vi "Demo of DBSCAN clustering.vi"() -> ()   [LabVIEW 2020]
doc: "Finds core samples of high density and expands clusters from them."
uses:
  Model/Unsupervised/Cluster/DBSCAN/Controls/dbscan_params.ctl
  Display/_Controls/Style.ctl
  Display/Classification/2D/Predicted/Controls/PredictedParameter.ctl
  Model/Unsupervised/Cluster/DBSCAN/DBSCAN.lvclass
  C:/Users/cipop/TDF Dropbox/2_Technologies de France/1 - Services et Etudes/PLAIY/2 - DEV/PLAIYLAB/code/Model/Model.lvclass
  Model/Unsupervised/Cluster/DBSCAN/DBSCAN.vi
  Preproc/Objet/3 - Model selection and evaluation/3.3 - Metrics and scoring/homogeneity_score/Homogeneity_Score.vi
  Preproc/Objet/3 - Model selection and evaluation/3.3 - Metrics and scoring/completeness_score/Completeness_Score.vi
  Preproc/Objet/3 - Model selection and evaluation/3.3 - Metrics and scoring/v_measure_score/V_Measure_Score.vi
  Preproc/Objet/3 - Model selection and evaluation/3.3 - Metrics and scoring/adjusted_rand_score/Adjusted_Rand_Score.vi
  Preproc/Objet/3 - Model selection and evaluation/3.3 - Metrics and scoring/adjusted_mutual_info_score/Adjusted_Mutual_Info_Score.vi
  Preproc/Objet/3 - Model selection and evaluation/3.3 - Metrics and scoring/silhouette_score/Silhouette_Score.vi
  Preproc/Objet/6 - Datasets Transformation/6.3 - Processing Data/StandardScaler/StandardScaler.lvclass
panel:
  in  "Local":T1
  in  "error in (no error) 2":errorcluster caption="entrée d'erreur (pas d'erreur)"
  out "Plot 2":cluster{"X":dbl[], "Y":dbl[]}[](graph) caption="Estimated number of cluster: 3"
  out "class_member_mask":bool[][](array[boolean])
  out "~core_samples_mask":bool[](array[boolean])
  out "n_noise_":i32
  out "error out":errorcluster
  out "Plot":cluster{"X":dbl[], "Y":dbl[]}[](graph) caption="Estimated number of cluster: 3"
  out "Silhouette Coefficient":string
  out "Adjusted Mutual Information":string
  out "Adjusted Rand Index":string
  out "V-measure":string
  out "Completeness":string
  out "Homogeneity":string
  out "n_clusters_":i32
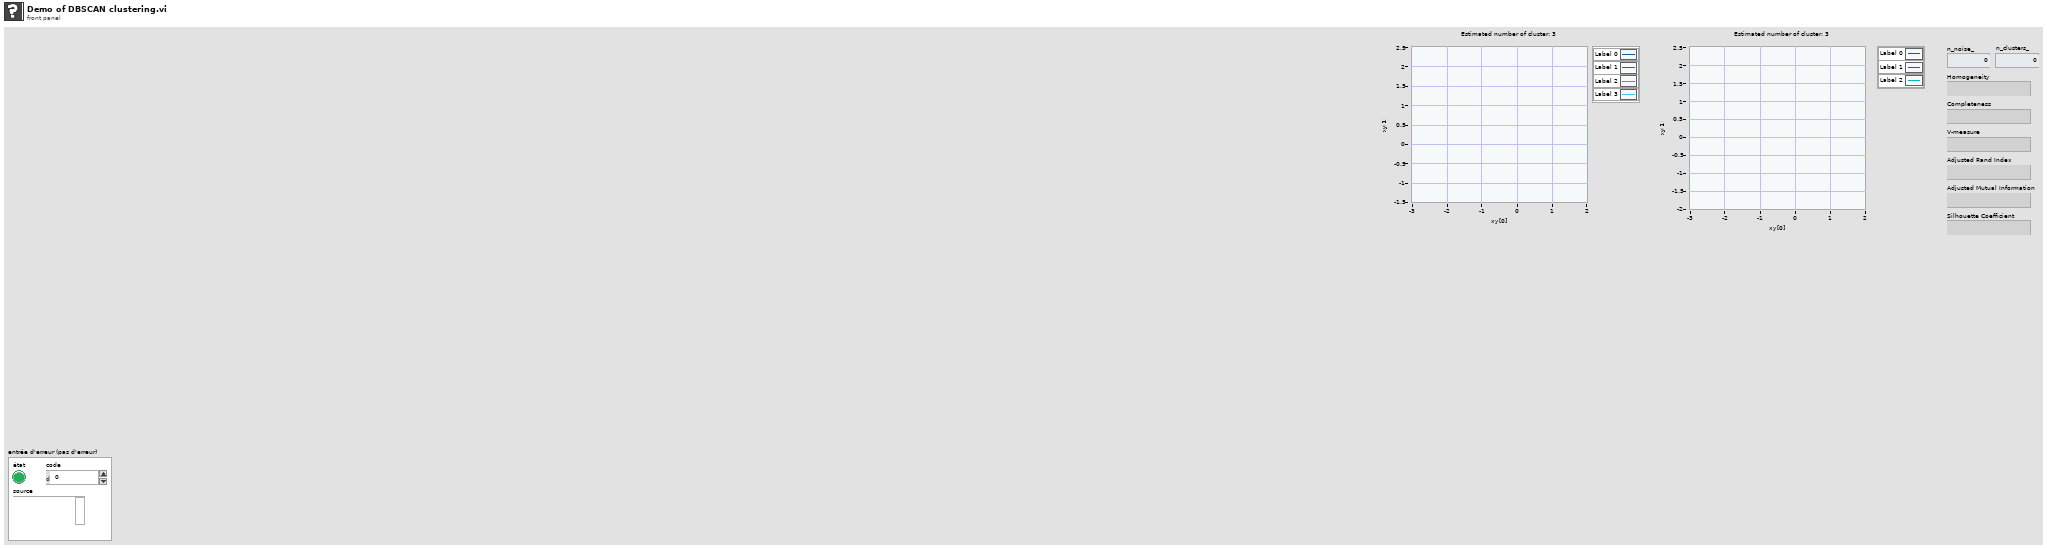
[diagram p1: front panel]
types:
  T1 = cluster{"X":dbl[][], "labels_true":dbl[], "core_sample_indices_":dbl[], "labels_":dbl[], "core_samples_mask":bool[], "Set_Label":dbl[], "1_Add_Mask":dbl[][], "2_Add_Mask":dbl[][], "1_Label_Add_Mask":dbl[][], "2_Label_Add_Mask":dbl[][]}
  T2 = cluster{"copy":bool, "with_mean":bool, "with_std":bool}
  T3 = cluster{"n_samples":i32[], "n_features":u32, "centers":i32[][], "cluster_std":dbl[], "centermin":dbl, "centermax":dbl, "shuffle":bool, "random_state":i32, "Returns":string}
  T4 = typedef "dbscan_params.ctl" = cluster{"eps":dbl, "min_samples":dbl, "metric":string, "algorithm":string, "leaf_size":dbl, "p":dbl, "n_jobs":dbl}
  T5 = typedef "Style.ctl" = enum16{"Empty circle", "Full circle", "Empty square", "Full square", "Cross"}
  T6 = typedef "PredictedParameter.ctl" = cluster{"Plot":refnum<vi>, "Data":cluster{"X":dbl[][], "Predict":dbl[][]}, "Indexe":cluster{"X":i32, "Y":i32}, "Point Property":cluster{"Style":T5, "Label Color":u32[]}}
  T7 = cluster{" 4DArray":cluster{"1":string[][], "2":string[][]}[], " 3DArray":cluster{"Tableau":string[][]}[], "Sparse Matrix 2DArray":string[][], " 2DArray":string[][], " 1DArray":string[]}
  T8 = typedef "dbscan_attributes.ctl" = cluster{"core_sample_indices_":dbl[], "components_":dbl[][], "labels_":dbl[]}
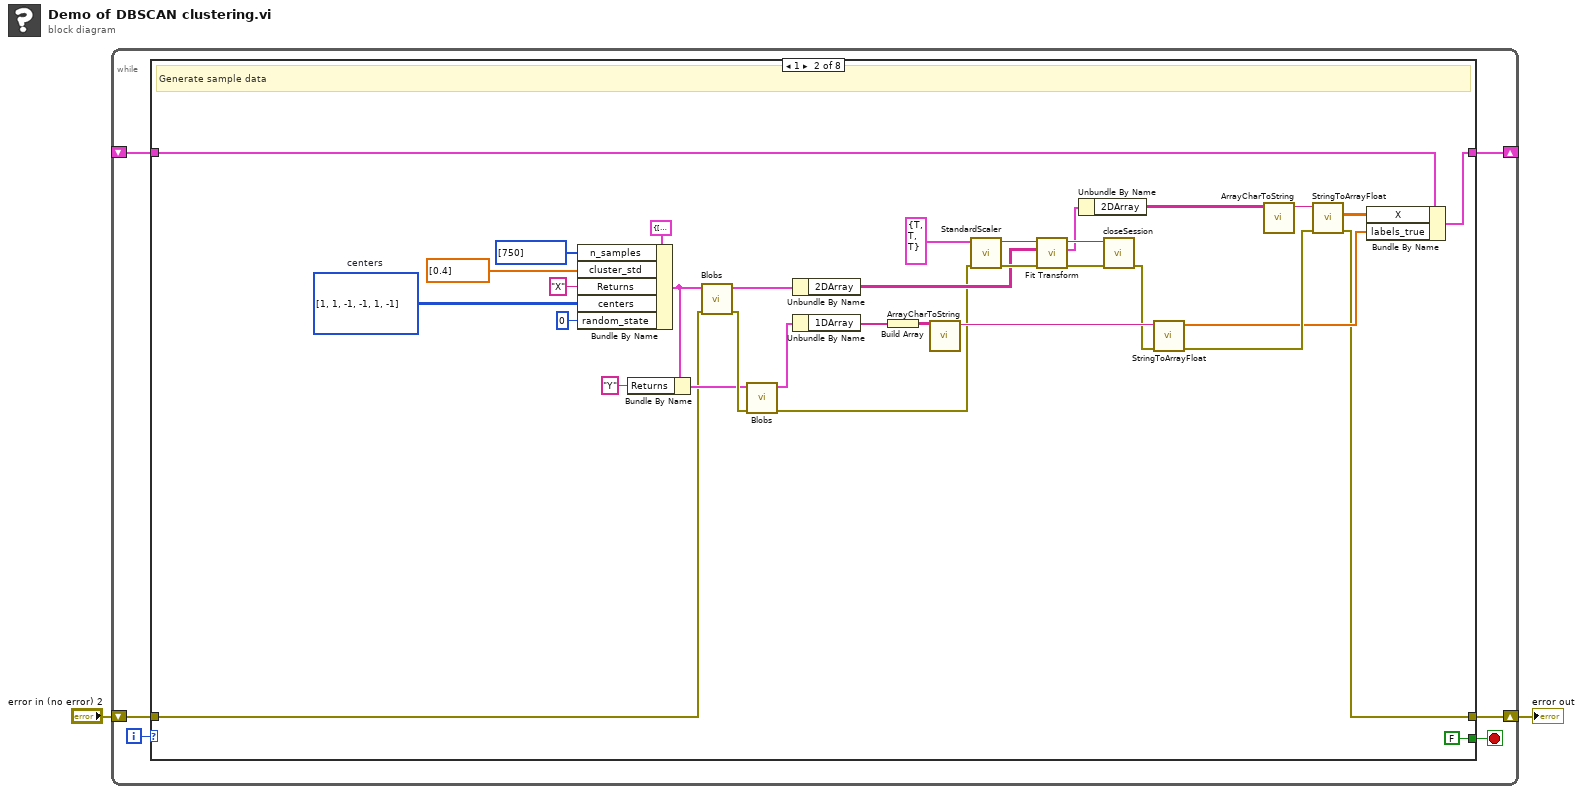
[diagram p0: block diagram]
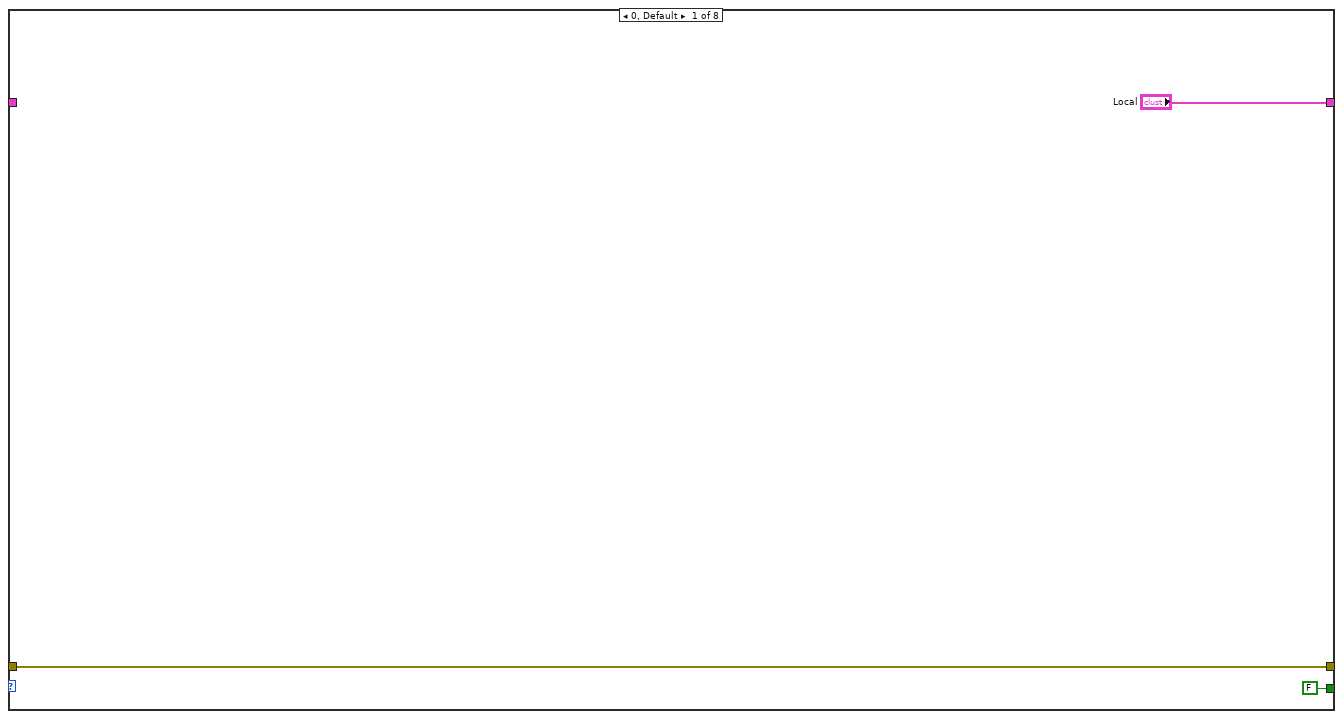
[diagram p2: hidden frame]
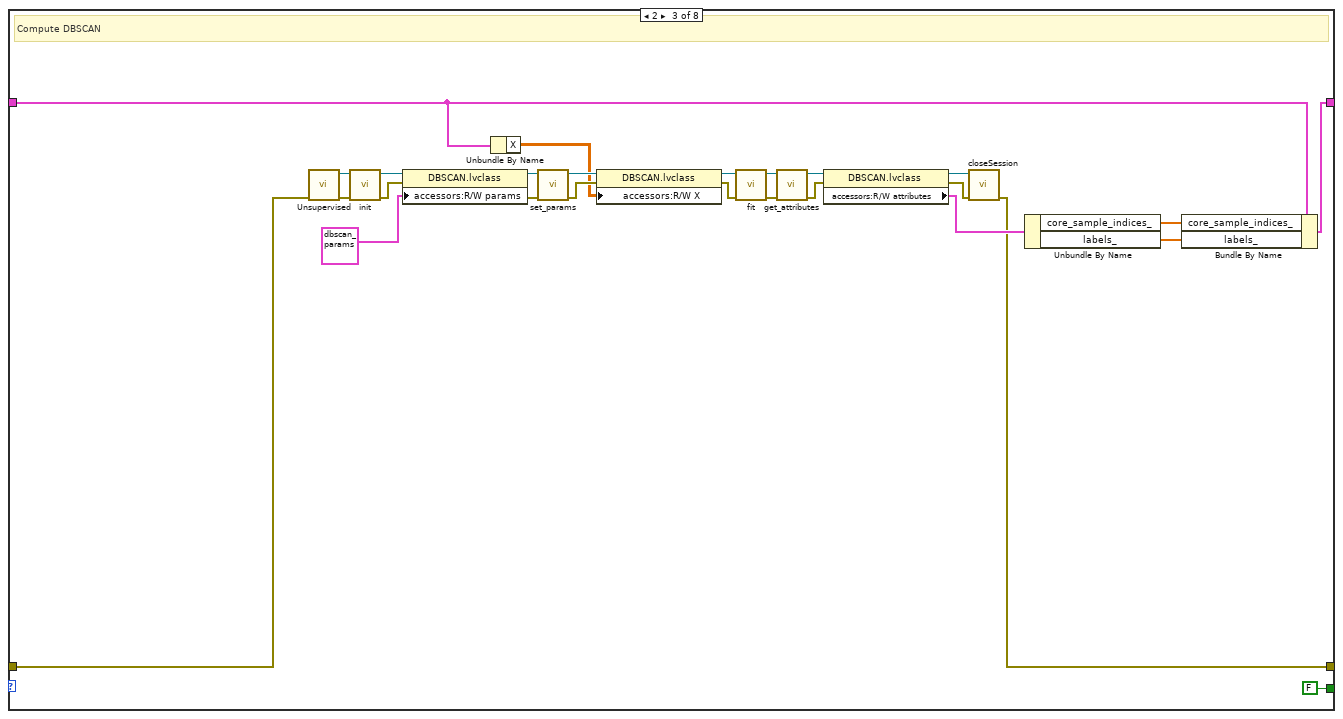
[diagram p3: hidden frame]
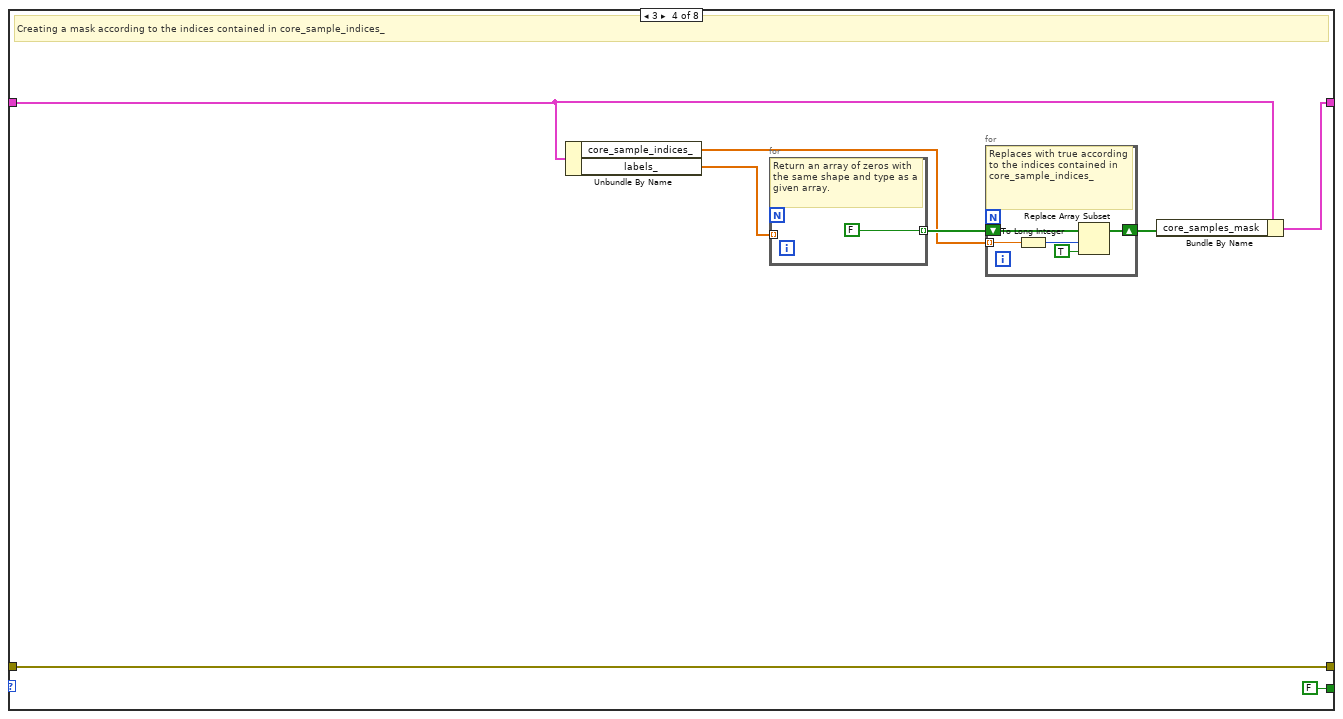
[diagram p4: hidden frame]
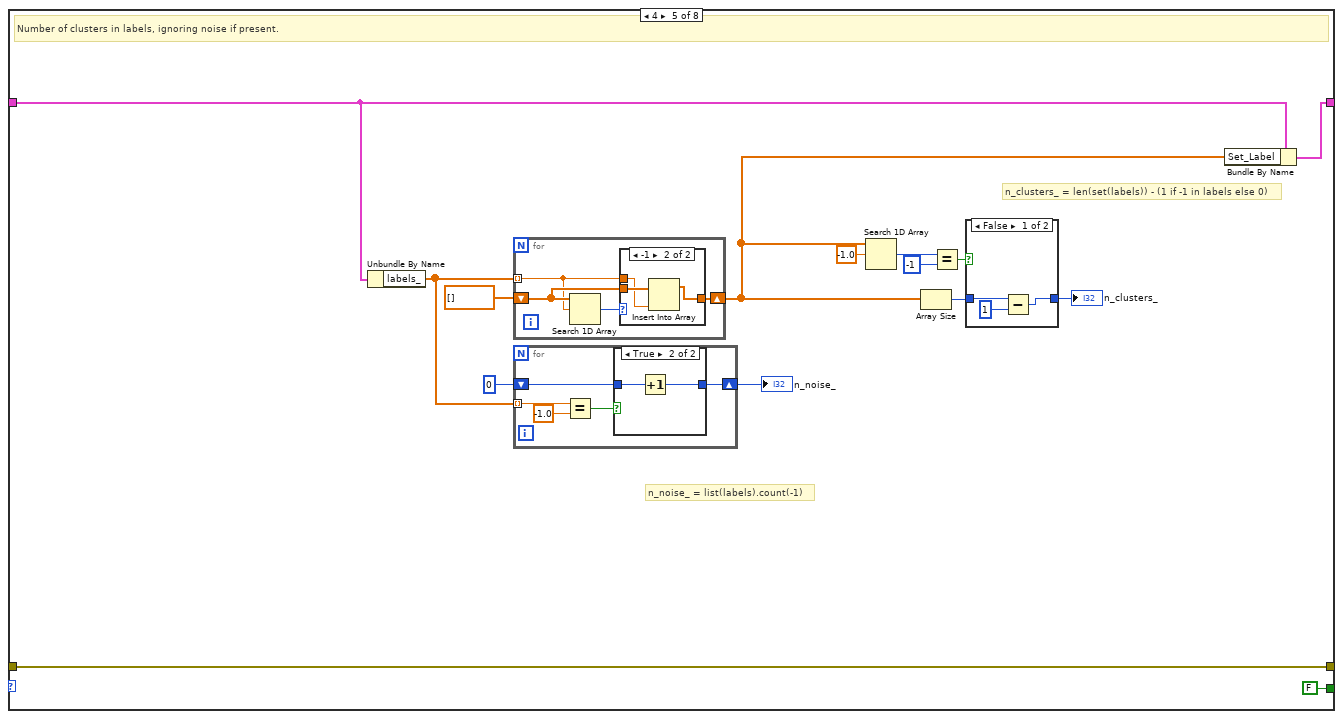
[diagram p5: hidden frame]
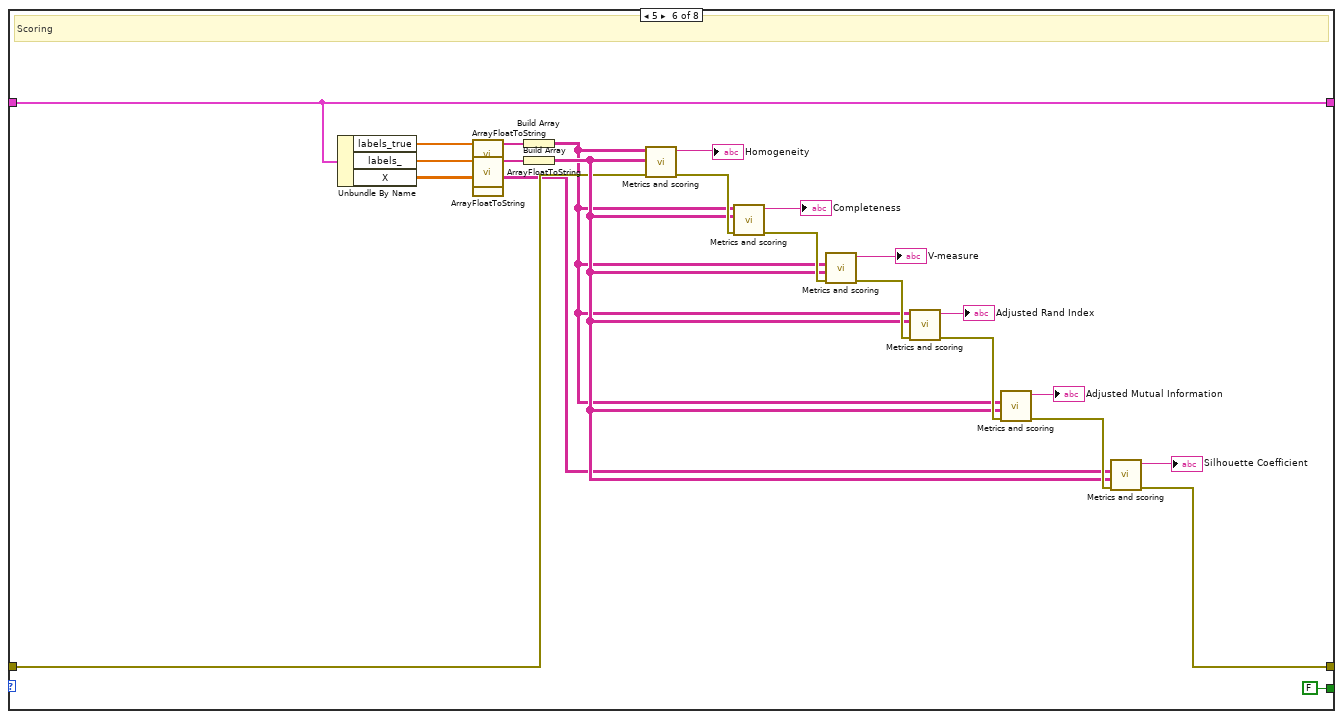
[diagram p9: hidden frame]
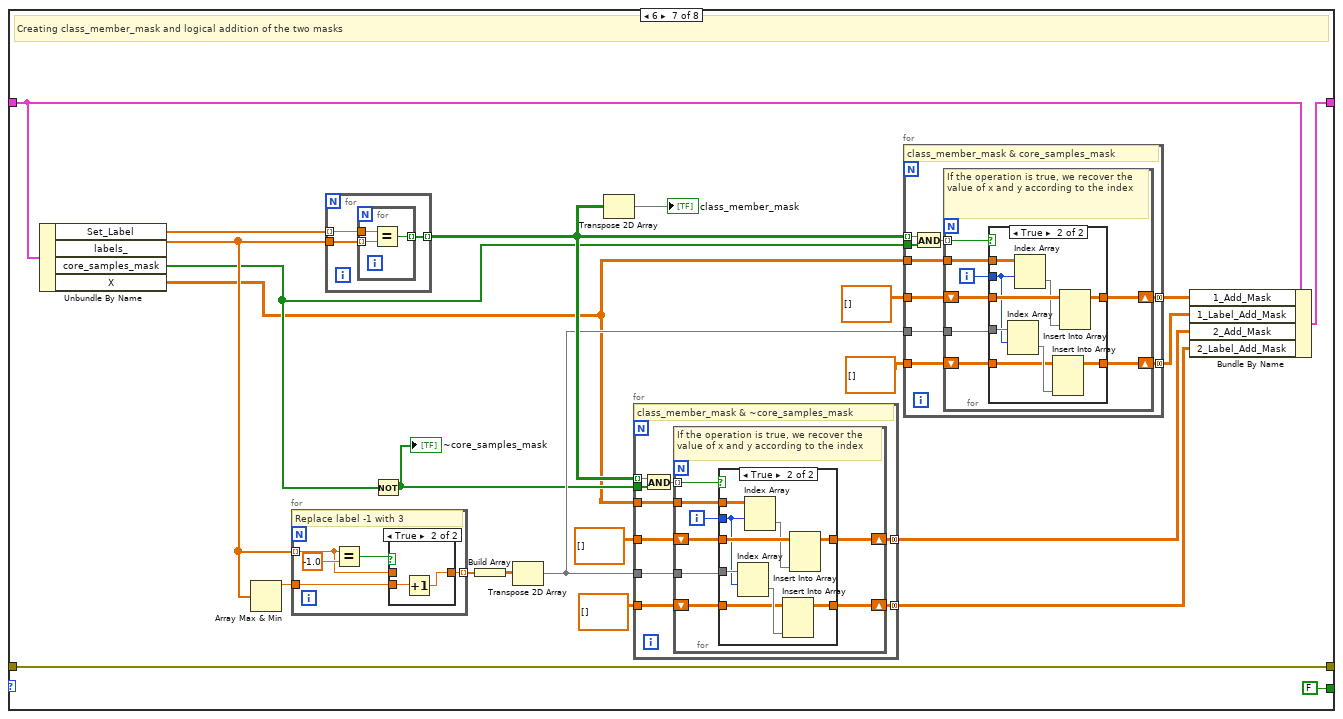
[diagram p10: hidden frame]
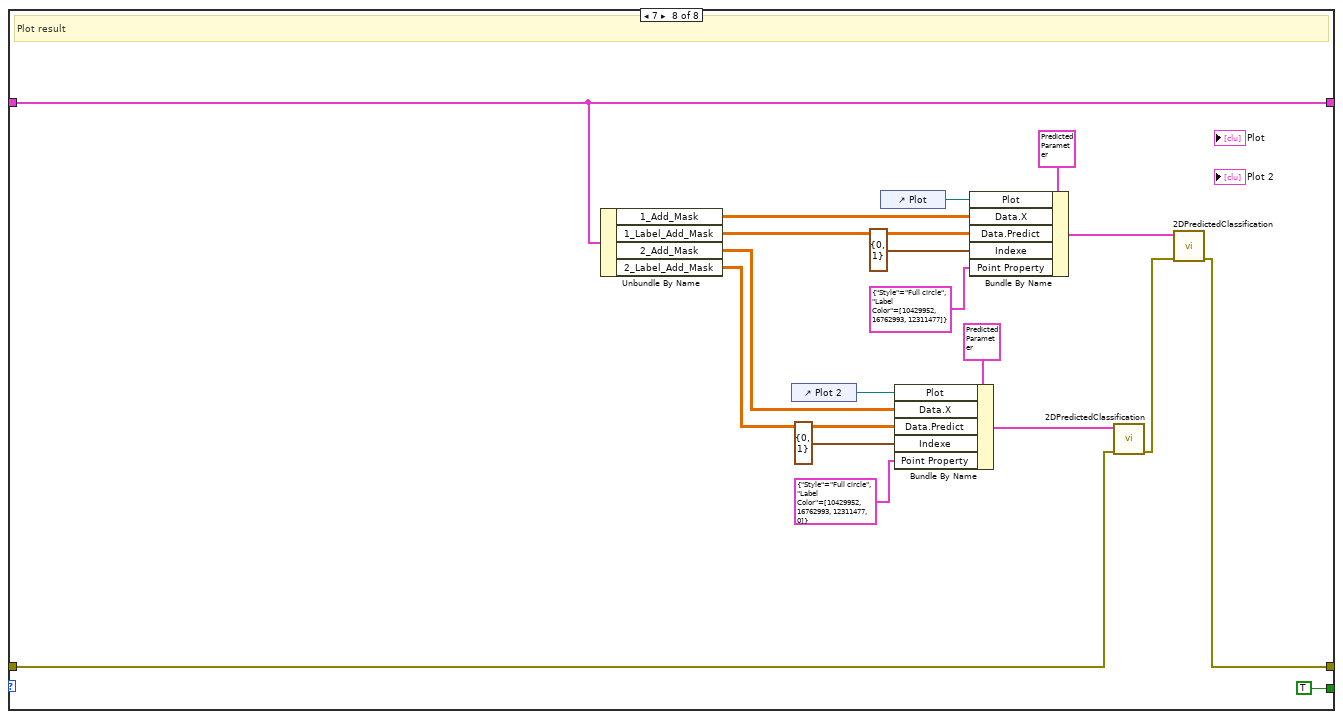
[diagram p14: hidden frame]
diagram:
  n1 = while {
    shift-right: [w3] -> _
    shift-left: _ -> [w7]
    shift-right: [w5] -> w1
    shift-left: "error in (no error) 2" -> [w6]
    i -> [w8]
    stop <- w4 stop-if-true
    n2 = case shown="1" w8 {
      tunnel: ["Local" w17 w53 w77 w93 w129 w150 w242] -> w3
      tunnel: w7 -> [_ w18 w49 w76 w88 w129 w151 w242]
      tunnel: w6 -> [w11 w13 w47 w73 w91 w127 w145 w245]
      tunnel: [w11 w14 w50 w73 w91 w136 w145 w246] -> w5
      tunnel: [FALSE FALSE FALSE FALSE FALSE FALSE FALSE TRUE] -> w4
      frame 0, Default {
      }
      frame 1 {
        w33 = i32[][] [[1, 1], [-1, -1], [1, -1]]  # centers
        # "Generate sample data"
        n3 = Bundle By Name(cluster=T3 {"n_samples"=[100], "n_features"=2, "centers"=[], "cluster_std"=[], "centermin"=-10.0, "centermax"=10.0, "shuffle"=TRUE, "random_state"=-1, "Returns"="X"} ("make_blobs"), "n_samples"=i32[] [750], "cluster_std"=dbl[] [0.4], "Returns"="X", "centers"=w33, "random_state"=0) -> (w31:T3)
        n4 = Bundle By Name(cluster=w31, "Returns"="Y") -> (w39:T3)
        n5 = call "Blobs.vi"("error in (no error)"=w13, "make_blobs"=w31) -> ("error out"=w43:errorcluster, "Data"=w45:T7)  [unwired: 8 in]
        n6 = call "Blobs.vi"("error in (no error)"=w43, "make_blobs"=w39) -> ("error out"=w23:errorcluster, "Data"=w38:T7)  [unwired: 8 in]
        n7 = Unbundle By Name(w45) -> ("2DArray"=w24:string[][])
        n8 = Unbundle By Name(w38) -> ("1DArray"=w35:string[])
        n9 = Build Array(w35) -> (w34:string[][])
        n10 = call "ArrayCharToString.vi"("TAB"=w34) -> ("Instruction"=w36:string)  [unwired: 10 in]
        n11 = call "StandardScaler.vi"("error in (no error)"=w23, "StandardScaler"=T2 {"copy"=TRUE, "with_mean"=TRUE, "with_std"=TRUE}) -> ("error out"=w25:errorcluster, "StandardScaler.lvclass"=w28:refnum<class "StandardScaler.lvclass">)  [unwired: 8 in]
        n12 = call-dynamic "Fit Transform.vi"("error in (no error)"=w25, "X"=w24, "StandardScaler.lvclass"=w28) -> ("error out"=w26:errorcluster, "Data"=w21:T7, "StandardScaler.lvclass"=w27:refnum<class "StandardScaler.lvclass">)  [unwired: 6 in]
        n13 = Unbundle By Name(w21) -> ("2DArray"=w20:string[][])
        n14 = call-dynamic "closeSession.vi"("error in"=w26, "Python en entrée"=w27) -> ("error out"=w22:errorcluster)  [unwired: 8 in, 1 out]
        n15 = call "StringToArrayFloat.vi"("entrée d'erreur (pas d'erreur)"=w22, "Return value"=w36) -> ("error IO"=w19:errorcluster, "1DArray"=w15:dbl[])  [unwired: 7 in, 1 out]
        n16 = call "ArrayCharToString.vi"("TAB"=w20) -> ("Instruction"=w44:string)  [unwired: 10 in]
        n17 = call "StringToArrayFloat.vi"("entrée d'erreur (pas d'erreur)"=w19, "Return value"=w44) -> ("error IO"=w14:errorcluster, "2DArray"=w16:dbl[][])  [unwired: 7 in, 1 out]
        n18 = Bundle By Name(cluster=w18, "X"=w16, "labels_true"=w15) -> (w17:T1)
      }
      frame 2 {
        # "Compute DBSCAN"
        n19 = call-poly "Unsupervised.vi"("error in"=w47) -> ("error out"=w70:errorcluster, "out"=w71:refnum<class "DBSCAN.lvclass">)  [unwired: 9 in]
        n20 = call-dynamic "init.vi"("error in (no error)"=w70, "Model en entrée"=w71) -> ("error out"=w62:errorcluster, "Model en sortie"=w66:refnum<class "DBSCAN.lvclass">)  [unwired: 8 in]
        n21 = property class="DBSCAN.lvclass"(reference=w66, error in=w62, "accessors:R/W params"=T4 {"eps"=0.3, "min_samples"=10.0, "metric"="euclidean", "algorithm"="auto", "leaf_size"=30.0, "p"=2.0, "n_jobs"=1.0} ("R/W params")) -> (reference out=w65:refnum<class "DBSCAN.lvclass">, error out=w67:errorcluster)
        n22 = Unbundle By Name(w49) -> ("X"=w48:dbl[][])
        n23 = call-dynamic "set_params.vi"("error in (no error)"=w67, "DBSCAN.lvclass 2"=w65) -> ("error out"=w63:errorcluster, "DBSCAN.lvclass"=w64:refnum<class "DBSCAN.lvclass">)  [unwired: 8 in]
        n24 = property class="DBSCAN.lvclass"(reference=w64, error in=w63, "accessors:R/W X"=w48) -> (reference out=w69:refnum<class "DBSCAN.lvclass">, error out=w68:errorcluster)
        n25 = call-dynamic "fit.vi"("error in (no error)"=w68, "DBSCAN.lvclass 2"=w69) -> ("error out"=w58:errorcluster, "DBSCAN.lvclass"=w59:refnum<class "DBSCAN.lvclass">)  [unwired: 8 in]
        n26 = call-dynamic "get_attributes.vi"("error in (no error)"=w58, "DBSCAN.lvclass 2"=w59) -> ("error out"=w56:errorcluster, "DBSCAN.lvclass"=w57:refnum<class "DBSCAN.lvclass">)  [unwired: 8 in]
        n27 = property class="DBSCAN.lvclass"(reference=w57, error in=w56) -> (reference out=w61:refnum<class "DBSCAN.lvclass">, error out=w60:errorcluster, "accessors:R/W attributes"=w55:T8)
        n28 = call-dynamic "closeSession.vi"("error in"=w60, "Python en entrée"=w61) -> ("error out"=w50:errorcluster)  [unwired: 8 in, 1 out]
        n29 = Unbundle By Name(w55) -> ("core_sample_indices_"=w52:dbl[], "labels_"=w51:dbl[])
        n30 = Bundle By Name(cluster=w49, "core_sample_indices_"=w52, "labels_"=w51) -> (w53:T1)
      }
      frame 3 {
        # "Creating a mask according to the indices contained in core_sample_indices_"
        n31 = Unbundle By Name(w76) -> ("core_sample_indices_"=w75:dbl[], "labels_"=w74:dbl[])
        n32 = for {
          tunnel: [FALSE] -> w79 mode=indexing
          tunnel: w74 -> [_] mode=indexing
          # "Return an array of zeros with the same shape and type as a given array."
        }
        n33 = for {
          tunnel: w75 -> [w84] mode=indexing
          shift-right: [w80] -> w78
          shift-left: w79 -> [w83]
          # "Replaces with true according to the indices contained in core_sample_indices_"
          n34 = To Long Integer(number=w84) -> (32bit integer=w82:i32)
          n35 = Replace Array Subset(array=w83, new element=TRUE ("new element/subarray"), index=w82) -> (w80:bool[])
        }
        n36 = Bundle By Name(cluster=w76, "core_samples_mask"=w78) -> (w77:T1)
      }
      frame 4 {
        # "n_noise_ = list(labels).count(-1)"
        # "n_clusters_ = len(set(labels)) - (1 if -1 in labels else 0)"
        # "Number of clusters in labels, ignoring noise if present."
        n37 = Unbundle By Name(w88) -> ("labels_"=w87:dbl[])
        n38 = for {
          tunnel: w87 -> [w114] mode=indexing
          shift-right: [w113] -> w92
          shift-left: dbl[] [] ("labels_") -> [w115]
          n39 = Search 1D Array(1D array=w115, element=w114) -> (index of element=w116:i32)  [unwired: 1 in]
          n40 = case shown="-1" w116 {
            tunnel: w115 -> [w117 w120]
            tunnel: w114 -> [_ w119]
            tunnel: [w117 w118] -> w113
            frame Default {
            }
            frame -1 {
              n41 = Insert Into Array(array=w120, new element=w119) -> (w118:dbl[])  [unwired: 1 in]
            }
          }
        }
        n42 = for {
          tunnel: w87 -> [w105] mode=indexing
          shift-right: [w102] -> w89
          shift-left: 0 -> [w101]
          n43 = Equal?(x=w105, y=-1.0) -> (x = y?=w103:bool)
          n44 = case shown="True" w103 {
            tunnel: [w106 w108] -> w102
            tunnel: w101 -> [w106 w107]
            frame False {
            }
            frame True {
              n45 = Increment(x=w107) -> (x+1=w108:i32)
            }
          }
        }
        "n_noise_" <- w89
        n46 = Search 1D Array(1D array=w92, element=-1.0) -> (index of element=w99:i32)  [unwired: 1 in]
        n47 = Array Size(array=w92) -> (size(s)=w98:i32)
        n48 = Equal?(x=w99, y=-1) -> (x = y?=w100:bool)
        n49 = case shown="False" w100 {
          tunnel: w98 -> [w111 w112]
          tunnel: [w109 w112] -> w90
          frame False {
            n50 = Subtract(x=w111, y=1) -> (x-y=w109:i32)
          }
          frame True {
          }
        }
        "n_clusters_" <- w90
        n51 = Bundle By Name(cluster=w88, "Set_Label"=w92) -> (w93:T1)
      }
      frame 5 {
        # "Scoring"
        n52 = Unbundle By Name(w129) -> ("labels_true"=w125:dbl[], "labels_"=w128:dbl[], "X"=w123:dbl[][])
        n53 = call "ArrayFloatToString.vi"("1D Data"=w125) -> ("Array"=w126:string[])  [unwired: 9 in, 1 out]
        n54 = call "ArrayFloatToString.vi"("1D Data"=w128) -> ("Array"=w142:string[])  [unwired: 9 in, 1 out]
        n55 = call "ArrayFloatToString.vi"("2D Data"=w123) -> ("Array"=w122:string[][])  [unwired: 9 in, 1 out]
        n56 = Build Array(w126) -> (w124:string[][])
        n57 = Build Array(w142) -> (w137:string[][])
        n58 = call-poly "Metrics and scoring.vi"("error in (no error)"=w127, "labels_pred"=w137, "labels_true"=w124) -> ("error out"=w143:errorcluster, "Score"=→"Homogeneity":string)  [unwired: 7 in]
        n59 = call-poly "Metrics and scoring.vi"("error in (no error)"=w143, "labels_pred"=w137, "labels_true"=w124) -> ("error out"=w141:errorcluster, "Score"=→"Completeness":string)  [unwired: 7 in]
        n60 = call-poly "Metrics and scoring.vi"("error in (no error)"=w141, "labels_pred"=w137, "labels_true"=w124) -> ("error out"=w140:errorcluster, "Score"=→"V-measure":string)  [unwired: 7 in]
        n61 = call-poly "Metrics and scoring.vi"("error in"=w140, "labels_pred"=w137, "labels_true"=w124) -> ("error out"=w139:errorcluster, "Score"=→"Adjusted Rand Index":string)  [unwired: 7 in]
        n62 = call-poly "Metrics and scoring.vi"("error in"=w139, "labels_pred"=w137, "labels_true"=w124) -> ("error out"=w138:errorcluster, "Score"=→"Adjusted Mutual Information":string)  [unwired: 7 in]
        n63 = call-poly "Metrics and scoring.vi"("error in (no error)"=w138, "labels"=w137, "X"=w122) -> ("error out"=w136:errorcluster, "Score"=→"Silhouette Coefficient":string)  [unwired: 7 in]
      }
      frame 6 {
        # "Creating class_member_mask and logical addition of the two masks"
        n64 = Unbundle By Name(w151) -> ("Set_Label"=w157:dbl[], "labels_"=w156:dbl[], "core_samples_mask"=w153:bool[], "X"=w152:dbl[][])
        n65 = Array Max & Min(array=w156) -> (max value=w165:dbl)  [unwired: 3 out]
        n66 = for {
          tunnel: w156 -> [w231] mode=indexing
          tunnel: [w230] -> w164 mode=indexing
          tunnel: w165 -> [w229]
          # "Replace label -1 with 3"
          n67 = Equal?(x=w231, y=-1.0) -> (x = y?=w232:bool)
          n68 = case shown="True" w232 {
            tunnel: w231 -> [w234 _]
            tunnel: [w234 w235] -> w230
            tunnel: w229 -> [_ w236]
            frame False {
            }
            frame True {
              n69 = Increment(x=w236) -> (x+1=w235:dbl)
            }
          }
        }
        n70 = for {
          tunnel: w156 -> [w225]
          tunnel: w157 -> [w224] mode=indexing
          tunnel: [w223] -> w159 mode=indexing
          n71 = for {
            tunnel: w225 -> [w228] mode=indexing
            tunnel: w224 -> [w227]
            tunnel: [w226] -> w223 mode=indexing
            n72 = Equal?(x=w227, y=w228) -> (x = y?=w226:bool)
          }
        }
        n73 = Not(x=w153) -> (.not. x?=w154:bool[])
        "~core_samples_mask" <- w154
        n74 = Build Array(w164) -> (w166:dbl[][])
        n75 = Transpose 2D Array(2D array=w166) -> (transposed array=w158:dbl[][])
        n76 = Transpose 2D Array(2D array=w159) -> (transposed array=→"class_member_mask":bool[][])
        n77 = for {
          tunnel: w159 -> [w203] mode=indexing
          tunnel: w154 -> [w202]
          tunnel: w152 -> [w200]
          tunnel: [w199] -> w147 mode=concatenating
          tunnel: dbl[][] [] ("2DArray") -> [w198]
          tunnel: w158 -> [w197]
          tunnel: [w195] -> w146 mode=concatenating
          tunnel: dbl[][] [] ("2DArray") -> [w196]
          # "class_member_mask & ~core_samples_mask"
          n78 = And(x=w203, y=w202) -> (x .and. y?=w201:bool[])
          n79 = for {
            tunnel: w201 -> [w210] mode=indexing
            tunnel: w200 -> [w211]
            shift-right: [w208] -> w199
            shift-left: w198 -> [w207]
            tunnel: w197 -> [w206]
            shift-right: [w204] -> w195
            shift-left: w196 -> [w205]
            i -> [w209]
            # "If the operation is true, we recover the value of x and y according to the index"
            n80 = case shown="True" w210 {
              tunnel: w211 -> [_ w222]
              tunnel: w209 -> [_ w214]
              tunnel: [w213 w219] -> w208
              tunnel: w207 -> [w213 w221]
              tunnel: w206 -> [_ w217]
              tunnel: w205 -> [w212 w216]
              tunnel: [w212 w215] -> w204
              frame False {
              }
              frame True {
                n81 = Index Array(array=w217, index (row)=w214) -> (element=w218:dbl[])  [unwired: 1 in]
                n82 = Index Array(array=w222, index (row)=w214) -> (element=w220:dbl[])  [unwired: 1 in]
                n83 = Insert Into Array(array=w216, new element=w218) -> (w215:dbl[][])  [unwired: 2 in]
                n84 = Insert Into Array(array=w221, new element=w220) -> (w219:dbl[][])  [unwired: 2 in]
              }
            }
          }
        }
        n85 = for {
          tunnel: w159 -> [w175] mode=indexing
          tunnel: w153 -> [w174]
          tunnel: w152 -> [w172]
          tunnel: [w171] -> w149 mode=concatenating
          tunnel: dbl[][] [] ("2DArray") -> [w170]
          tunnel: w158 -> [w169]
          tunnel: [w167] -> w148 mode=concatenating
          tunnel: dbl[][] [] ("2DArray") -> [w168]
          # "class_member_mask & core_samples_mask"
          n86 = And(x=w175, y=w174) -> (x .and. y?=w173:bool[])
          n87 = for {
            tunnel: w173 -> [w182] mode=indexing
            tunnel: w172 -> [w183]
            shift-right: [w180] -> w171
            shift-left: w170 -> [w179]
            tunnel: w169 -> [w178]
            shift-right: [w176] -> w167
            shift-left: w168 -> [w177]
            i -> [w181]
            # "If the operation is true, we recover the value of x and y according to the index"
            n88 = case shown="True" w182 {
              tunnel: w183 -> [_ w194]
              tunnel: w181 -> [_ w186]
              tunnel: [w185 w191] -> w180
              tunnel: w179 -> [w185 w193]
              tunnel: w178 -> [_ w189]
              tunnel: w177 -> [w184 w188]
              tunnel: [w184 w187] -> w176
              frame False {
              }
              frame True {
                n89 = Index Array(array=w189, index (row)=w186) -> (element=w190:dbl[])  [unwired: 1 in]
                n90 = Index Array(array=w194, index (row)=w186) -> (element=w192:dbl[])  [unwired: 1 in]
                n91 = Insert Into Array(array=w188, new element=w190) -> (w187:dbl[][])  [unwired: 2 in]
                n92 = Insert Into Array(array=w193, new element=w192) -> (w191:dbl[][])  [unwired: 2 in]
              }
            }
          }
        }
        n93 = Bundle By Name(cluster=w151, "1_Add_Mask"=w149, "1_Label_Add_Mask"=w148, "2_Add_Mask"=w147, "2_Label_Add_Mask"=w146) -> (w150:T1)
      }
      frame 7 {
        # "Plot result"
        n94 = Unbundle By Name(w242) -> ("1_Add_Mask"=w241:dbl[][], "1_Label_Add_Mask"=w240:dbl[][], "2_Add_Mask"=w239:dbl[][], "2_Label_Add_Mask"=w238:dbl[][])
        n95 = control-ref of="Plot 2"() -> (w243:refnum<vi>)
        n96 = control-ref of="Plot"() -> (w244:refnum<vi>)
        n97 = Bundle By Name(cluster=T6 {"Plot"=refnum, "Data"={"X"=[], "Predict"=[]}, "Indexe"={"X"=0, "Y"=1}, "Point Property"={"Style"=enum."Full circle", "Label Color"=[8978528, 4367871, 1985280]}} ("Parameters"), "Plot"=w243, "Data.X"=w239, "Data.Predict"=w238, "Indexe"=cluster{"X":i32, "Y":i32} {"X"=0, "Y"=1}, "Point Property"=cluster{"Style":T5, "Label Color":u32[]} {"Style"=enum."Full circle", "Label Color"=[10429952, 16762993, 12311477, 0]}) -> (w254:T6)
        n98 = Bundle By Name(cluster=T6 {"Plot"=refnum, "Data"={"X"=[], "Predict"=[]}, "Indexe"={"X"=0, "Y"=1}, "Point Property"={"Style"=enum."Full circle", "Label Color"=[8978528, 4367871, 1985280]}} ("Parameters"), "Plot"=w244, "Data.X"=w241, "Data.Predict"=w240, "Indexe"=cluster{"X":i32, "Y":i32} {"X"=0, "Y"=1}, "Point Property"=cluster{"Style":T5, "Label Color":u32[]} {"Style"=enum."Full circle", "Label Color"=[10429952, 16762993, 12311477]}) -> (w249:T6)
        n99 = call "2DPredictedClassification.vi"("error in"=w245, "Parameters"=w254) -> ("error out"=w247:errorcluster)  [unwired: 9 in]
        n100 = call "2DPredictedClassification.vi"("error in"=w247, "Parameters"=w249) -> ("error out"=w246:errorcluster)  [unwired: 9 in]
      }
    }
  }
  "error out" <- w1
